vi "Wait for Obtain.vi"(8 "error in (no error)":errorcluster, 9 "ms Timeout (5000)":u32=5000, 11 "Queue Name":string) -> (0 "error out":errorcluster, 1 "ms Elapsed":u32, 3 "Queue out":refnum<queue>)   [LabVIEW 2021, in "Queue.lvlib"]
doc: "Wait for a named queue to be created. Rather than assuming a queue will be created, this waits for the child thread to create the queue. In multi-threaded applications, sub-threads may not be created at Run-Time, this ensures the thread that owns the queue reference is responsible for creating and destroying the queue reference. Specify the <b>ms Timeout</b> to limit the time to wait for the <b>Queue Name</b> to be obtained."
uses:
  Queue.lvlib
  <vilib>/Utility/error.llb/Error Cluster From Error Code.vi
  <vilib>/ErrorRing/Error Ring.xnode
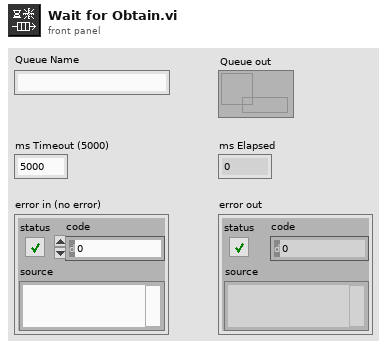
[diagram p1: front panel]
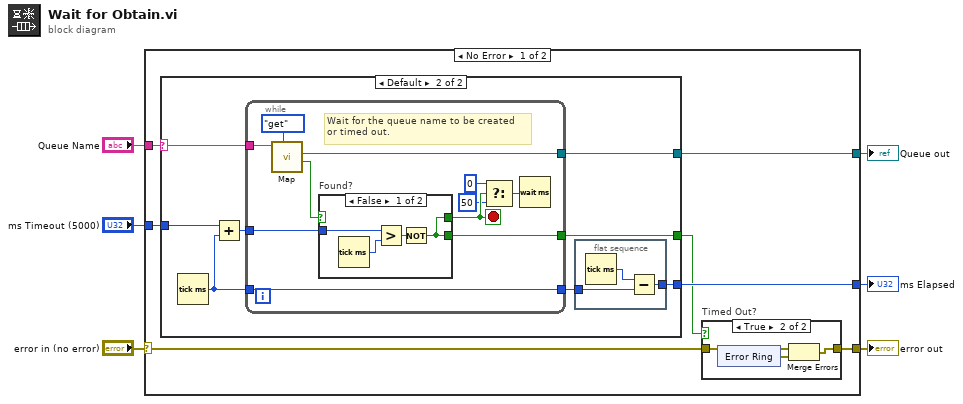
[diagram p0: block diagram]
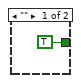
[diagram p3: hidden frame]
diagram:
  n1 = case shown="No Error" "error in (no error)" {
    selector: "error in (no error)" -> [w10 w50]
    tunnel: "Queue Name" -> [w13 _]
    tunnel: "ms Timeout (5000)" -> [w12 _]
    tunnel: [w11 _] -> w4
    tunnel: [w9 w50] -> w2
    tunnel: [w8 _] -> w1
    frame No Error {
      n2 = case shown="Default" w13 {
        selector: w13 -> [_ w30]
        tunnel: w12 -> [_ w29]
        tunnel: [_ w28] -> w11
        tunnel: [_ w26] -> w8
        tunnel: [TRUE w23] -> w7
        frame "" {
        }
        frame Default {
          n3 = Tick Count (ms)() -> (millisecond timer value=w25:u32)
          n4 = Add(x=w29, y=w25) -> (x+y=w27:u32)
          n5 = while {
            tunnel: w30 -> [w43]
            tunnel: [w42] -> w28
            tunnel: w27 -> [w40]
            tunnel: [w38] -> w23
            tunnel: [w34] -> w24
            tunnel: w25 -> [w34]
            stop <- w36 stop-if-true
            # "Wait for the queue name to be created\nor timed out."
            n6 = call "Map.vi"("Action"=enum8{"noop", "get", "set", "pop"}."get", "Queue Name"=w43) -> ("Found?"=w41:bool, "Queue out"=w42:refnum<queue>)  [unwired: 7 in, 1 out]
            n7 = case "Found?" shown="False" w41 {
              selector: w41 -> [_ w49]
              tunnel: w40 -> [w48 _]
              tunnel: [w45 _] -> w38
              tunnel: [w45 w49] -> w36
              frame False {
                n8 = Tick Count (ms)() -> (millisecond timer value=w47:u32)
                n9 = Greater?(x=w48, y=w47) -> (0:w46:bool)
                n10 = Not(x=w46) -> (.not. x?=w45:bool)
              }
              frame True {
              }
            }
            n11 = Select(t=u32 0 ("milliseconds to wait"), s=w36, f=u32 50 ("milliseconds to wait")) -> (s? t:f=w37:u32)
            n12 = Wait (ms)(milliseconds to wait=w37) -> ()  [unwired: 1 out]
          }
          n13 = flat-sequence {
            tunnel: w24 -> [w32]
            tunnel: [w31] -> w26
            frame #0 {
              n14 = Tick Count (ms)() -> (millisecond timer value=w33:u32)
              n15 = Subtract(x=w33, y=w32) -> (x-y=w31:u32)
            }
          }
        }
      }
      n16 = case "Timed Out?" shown="True" w7 {
        tunnel: w10 -> [w14 w17]
        tunnel: [w14 w16] -> w9
        frame False {
        }
        frame True {
          n17 = xnode "Error Ring"() -> ("error out"=w15:errorcluster)
          n18 = Merge Errors(w17, w15) -> (w16:errorcluster)
        }
      }
    }
    frame Error {
    }
  }
  "error out" <- w2
  "Queue out" <- w4
  "ms Elapsed" <- w1
